vi "st_str Acquire Data from Hardware(forSubVi).vi"(8 "error in (no error)":errorcluster, 11 "GenParametr":T1={"UgenVrms"=0.0, "Frequency 1,kHz"=0.0, "dFreq, kHz"=0.0, "Frequency 2,kHz"=0.0, "WaitSignalGen"=150.0}) -> (0 "error out":errorcluster, 3 "AllParametrArray":dbl[][](array[numeric]))   [LabVIEW 2017]
doc: "Generates sample waveforms according to the signal type in the HW Config input."
uses:
  controls/st_str gen parametr.ctl
  st_voltmetr/subVIs/st_str Global.vi
panel:
  out "Protocol":string[][](table)
  in  "StopAcquire":bool
  out "V":dbl[](array[numeric])
  out "WaitSignalGen":u32=150
  out "ChangeGenParam":bool
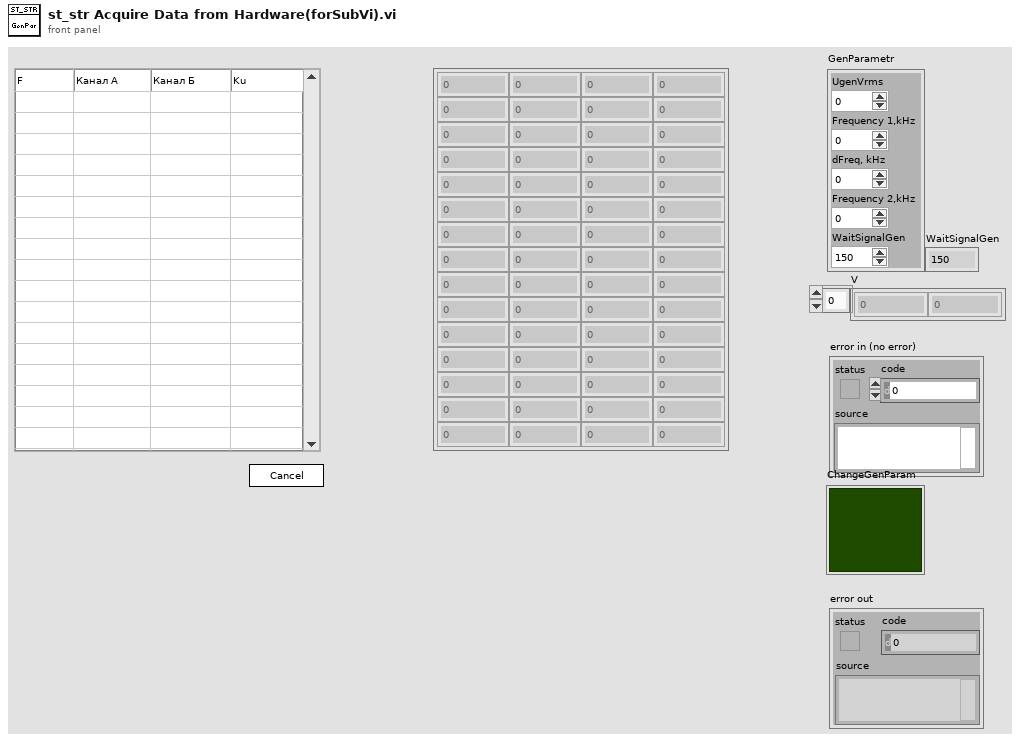
[diagram p1: front panel]
types:
  T1 = typedef "st_str gen parametr.ctl" = cluster{"UgenVrms":dbl, "Frequency 1,kHz":dbl, "dFreq, kHz":dbl, "Frequency 2,kHz":dbl, "WaitSignalGen":dbl}
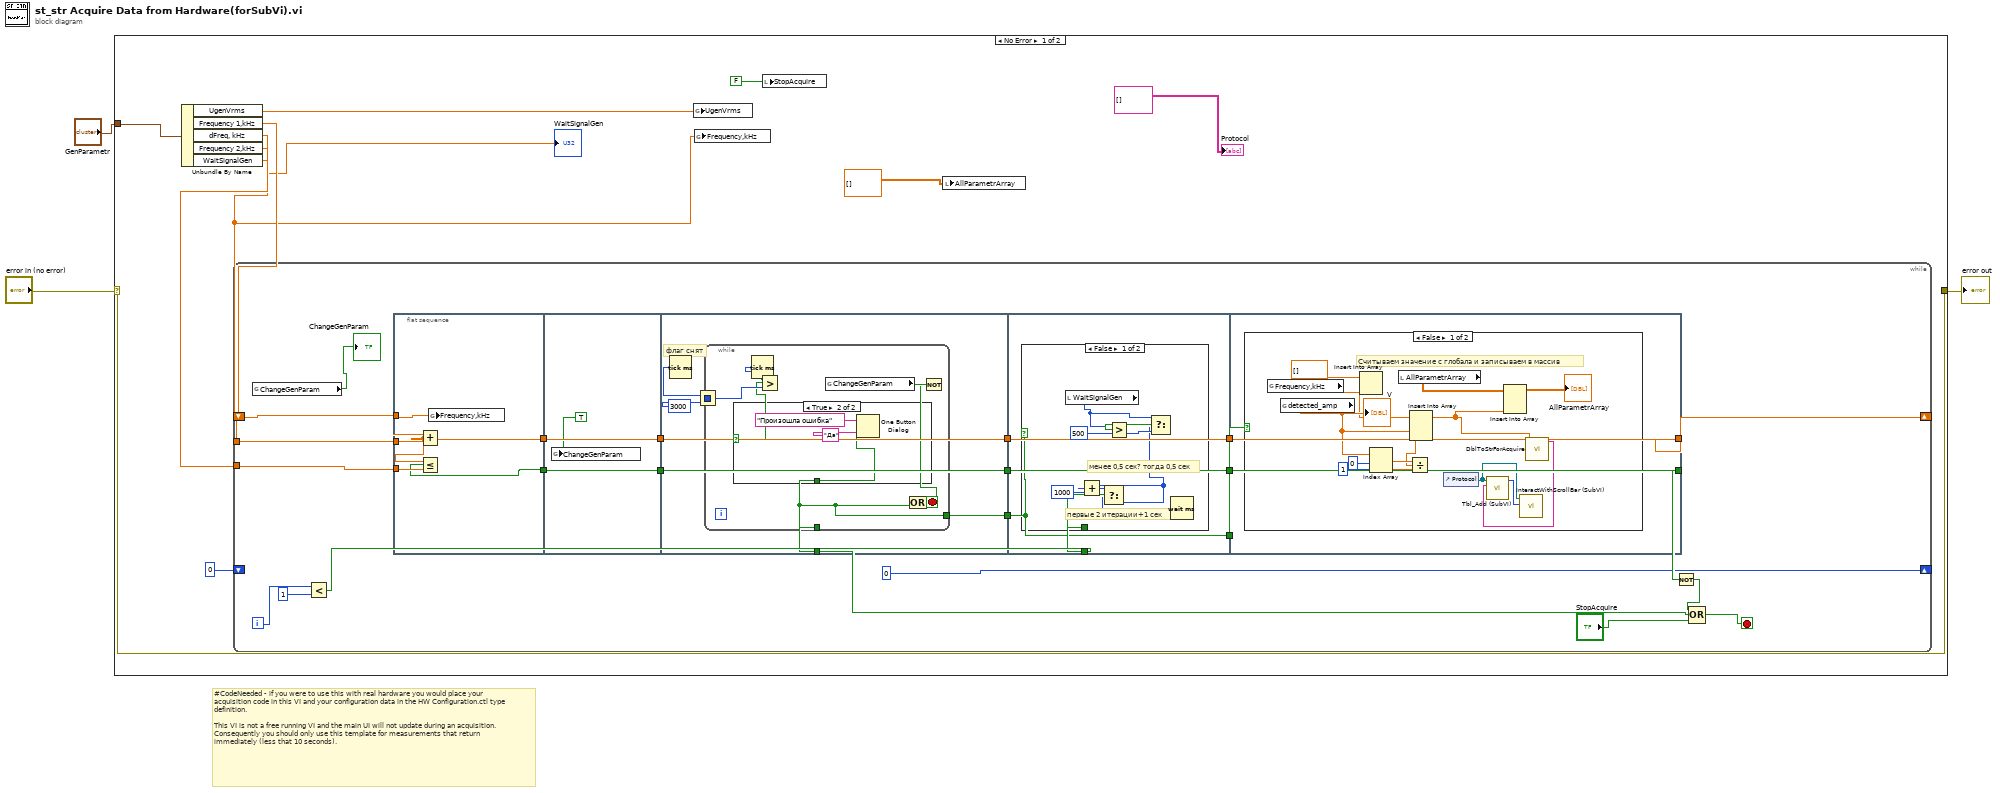
[diagram p0: block diagram]
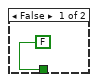
[diagram p2: hidden frame]
diagram:
  # "#CodeNeeded - if you were to use this with real hardware you would place your acquisition code in this VI and your configuration data in the HW Configuration.ctl type definition.\n\nThis VI is not a free running VI and the main UI will not update during an acquisition.  Consequently you should only use this template for measurements that return immediately (less that 10 seconds)."
  n1 = case shown="No Error" "error in (no error)" {
    selector: "error in (no error)" -> [w14 w95]
    tunnel: [w14 w95] -> w2
    tunnel: "GenParametr" -> [w13 _]
    frame No Error {
      n2 = Unbundle By Name(w13) -> ("UgenVrms"=w6:dbl, "Frequency 1,kHz"=w10:dbl, "dFreq, kHz"=w7:dbl, "Frequency 2,kHz"=w9:dbl, "WaitSignalGen"=→"WaitSignalGen":dbl)
      n3 = while {
        shift-right: [w37] -> _
        shift-left: w10 -> [w35]
        tunnel: w7 -> [w38]
        tunnel: w9 -> [w36]
        shift-right: [0] -> _
        shift-left: 0 -> [_]
        i -> [w29]
        stop <- w31 stop-if-true
        # "флаг снят"
        n4 = global read "st_str Global.vi" "ChangeGenParam"() -> (→"ChangeGenParam":bool)
        n5 = Less?(x=w29, y=1) -> (x < y?=w27:bool)
        n6 = flat-sequence {
          tunnel: w38 -> [w43]
          tunnel: w36 -> [w41]
          tunnel: w35 -> [w39]
          tunnel: [w42] -> w26
          tunnel: [w40] -> w25
          tunnel: w26 -> [w46]
          tunnel: w25 -> [w45]
          tunnel: [w46] -> w22
          tunnel: [w45] -> w20
          tunnel: w22 -> [w53]
          tunnel: [w53] -> w21
          tunnel: w20 -> [w52]
          tunnel: [w52] -> w19
          tunnel: [w48] -> w18
          tunnel: [w47] -> w16
          tunnel: w21 -> [w68]
          tunnel: [w68] -> w24
          tunnel: w19 -> [w67]
          tunnel: [w67] -> w23
          tunnel: w27 -> [w66]
          tunnel: w16 -> [w65]
          tunnel: [w65] -> w15
          tunnel: [w78] -> w34
          tunnel: [w79] -> w37
          tunnel: w24 -> [w79]
          tunnel: w23 -> [w78]
          tunnel: w15 -> [w77]
          frame #0 {
            n7 = Add(x=w39, y=w43) -> (x+y=w42:dbl)
            n8 = Less Or Equal?(x=w42, y=w41) -> (x <= y?=w40:bool)
            n9 = global write "st_str Global.vi" "Frequency,kHz"(w39) -> ()
          }
          frame #1 {
            n10 = global write "st_str Global.vi" "ChangeGenParam"(TRUE ("ChangeGenParam")) -> ()
          }
          frame #2 {
            n11 = Tick Count (ms)() -> (millisecond timer value=w51:u32)
            n12 = Add(x=w51, y=u32 3000) -> (x+y=w49:u32)
            n13 = while {
              tunnel: w49 -> [w59]
              tunnel: [w54] -> w48
              tunnel: [w54] -> w47
              stop <- w56 stop-if-true
              n14 = Tick Count (ms)() -> (millisecond timer value=w60:u32)
              n15 = Greater?(x=w60, y=w59) -> (0:w58:bool)
              n16 = case shown="True" w58 {
                tunnel: [FALSE ("true") w62] -> w54
                frame False {
                }
                frame True {
                  n17 = One Button Dialog(message="Произошла ошибка", button name ("OK")="Да") -> (true=w62:bool)
                }
              }
              n18 = global read "st_str Global.vi" "ChangeGenParam"() -> (w57:bool)
              n19 = Not(x=w57) -> (.not. x?=w55:bool)
              n20 = Compound Arithmetic op=OR(w55, w54) -> (w56:bool)
            }
          }
          frame #3 {
            n21 = case shown="False" w65 {
              tunnel: w66 -> [w73 _]
              frame False {
                w74 = u32 500 ("y")
                # "первые 2 итерации+1 сек"
                # "менее 0,5 сек? тогда 0,5 сек"
                n22 = local read "WaitSignalGen"() -> (w75:u32)
                n23 = Greater?(x=w75, y=w74) -> (0:w76:bool)
                n24 = Select(t=w75, s=w76, f=w74) -> (s? t:f=w71:u32)
                n25 = Add(x=w71, y=u32 1000) -> (x+y=w72:u32)
                n26 = Select(t=w72, s=w73, f=w71) -> (s? t:f=w69:u32)
                n27 = Wait (ms)(milliseconds to wait=w69) -> ()  [unwired: 1 out]
              }
              frame True {
              }
            }
          }
          frame #4 {
            n28 = case shown="False" w77 {
              frame False {
                # "Считываем значение с глобала и записываем в массив"
                n29 = global read "st_str Global.vi" "Frequency,kHz"() -> (w86:dbl)
                n30 = global read "st_str Global.vi" "detected_amp"() -> (w88:dbl[])
                "V" <- w88
                n31 = Insert Into Array(array=dbl[] [], new element=w86) -> (w85:dbl[])  [unwired: 1 in]
                n32 = Index Array(array=w88, index #1=0 ("index"), index #2=1 ("index")) -> (element #1=w90:dbl, element #2=w91:dbl)
                n33 = local read "AllParametrArray"() -> (w94:dbl[][])
                n34 = Divide(x=w90, y=w91) -> (x/y=w89:dbl)
                n35 = Insert Into Array(array=w85, new element #1=w88, new element #2=w89) -> (w81:dbl[])  [unwired: 1 in]
                n36 = control-ref of="Protocol"() -> (w83:refnum<vi>)
                n37 = Insert Into Array(array=w94, new element=w81) -> (→"AllParametrArray":dbl[][])  [unwired: 2 in]
                n38 = call "DblToStrForAcquire.vi"("DataDbl"=w81) -> ("Out"=w80:string[])  [unwired: 10 in]
                n39 = call "Tbl_Add (SubVI).vi"("meas"=w80, "Table in"=w83) -> ("element"=w82:i32)  [unwired: 9 in]
                n40 = call "InteractWithScrollBar (SubVI).vi"("element"=w82, "Table in"=w83) -> ()  [unwired: 10 in]
              }
              frame True {
              }
            }
          }
        }
        n41 = Not(x=w34) -> (.not. x?=w33:bool)
        n42 = Compound Arithmetic op=OR(w33, w18, "StopAcquire") -> (w31:bool)
      }
      n43 = global write "st_str Global.vi" "UgenVrms"(w6) -> ()
      n44 = global write "st_str Global.vi" "Frequency,kHz"(w7) -> ()
      n45 = local write "StopAcquire"(FALSE ("StopAcquire")) -> ()
      n46 = local write "AllParametrArray"(dbl[][] []) -> ()
      "Protocol" <- string[][] []
    }
    frame Error {
    }
  }
  "error out" <- w2
